vi "Main.vi"() -> ()   [LabVIEW 2023]
uses:
  <vilib>/userDefined/High Color/IMAQdx.ctl
  <vilib>/vision/Image Controls.llb/IMAQ Image.ctl
  <vilib>/vision/driver/NI_Vision_Acquisition_Software.lvlib
  <resource>/objmgr/imaqdx.rc
panel:
  out "New Image":T1
  in  "Object Parameters Attributes":T2={"ReflectedTemperature"=300.0, "AtmosphericTemperature"=300.0, "ExtOpticsTemperature"=300.0, "ObjectEmissivity "=0.95, "RelativeHumidity "=1.0, "ExtOpticsTransmission"=1.0, "EstimatedTransmission"=0.0, "ObjectDistance"=0.0} {"ObjectDistance" min=0.0 max=10000.0 step=1.0; "EstimatedTransmission" min=0.0 max=1.0 step=0.01; "ExtOpticsTransmission" min=0.0 max=1.0 step=0.01; "RelativeHumidity" min=0.0 max=1.0 step=0.01; "ObjectEmissivity" min=0.0 max=1.0 step=0.01; "ExtOpticsTemperature" min=0.0 max=5000.0 step=1.0; "AtmosphericTemperature" min=0.0 max=5000.0 step=1.0; "ReflectedTemperature" min=0.0 max=5000.0 step=1.0}
  in  "PacketSize":u32=1500
  in  "NUCMode":enum16{"Off", "On"}(ring)=enum."On"
  in  "IRFormat":i64(ring)=1 items=["Radiometric", "TemperatureLinear100mK", "TemperatureLinear10mK"]
  in  "Session In":T3
  out "Temperature":dbl(slide) scale=24.600000000000023..25.400000000000034
  out "Image":T1(plugin-control)
  in  "Stop":bool
  # "Please select the camera you want to access the thermal image"
  # "Note: The Image control needs to be set to 16-bit display. This is done by with the following steps\n            1) Right click on the Image display and select 16-Bit Display Mapping to bring up Set 16 Bit Display Mapping window\n            2) Un-tick \"Apply mapping only when Configured bit depth is 0\" in the Set 16 Bit Display Mapping window\n            3) Set the Conversion Method to Full Dynamic if not already selected"
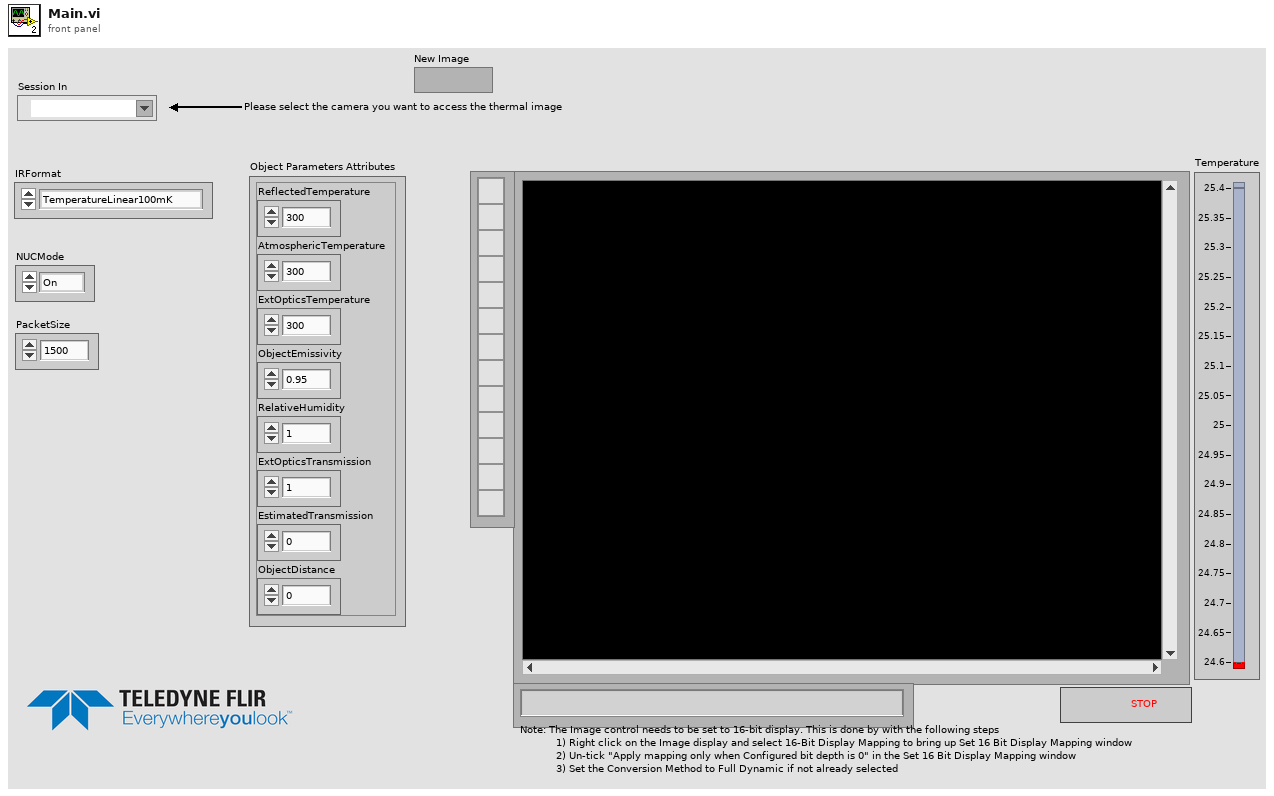
[diagram p1: front panel]
types:
  T1 = typedef "IMAQ Image.ctl" = refnum<image>
  T2 = cluster{"ReflectedTemperature":dbl, "AtmosphericTemperature":dbl, "ExtOpticsTemperature":dbl, "ObjectEmissivity ":dbl, "RelativeHumidity ":dbl, "ExtOpticsTransmission":dbl, "EstimatedTransmission":dbl, "ObjectDistance":dbl}
  T3 = typedef "IMAQdx.ctl" = refnum<k21>
  T4 = typedef "Image Type" = u32
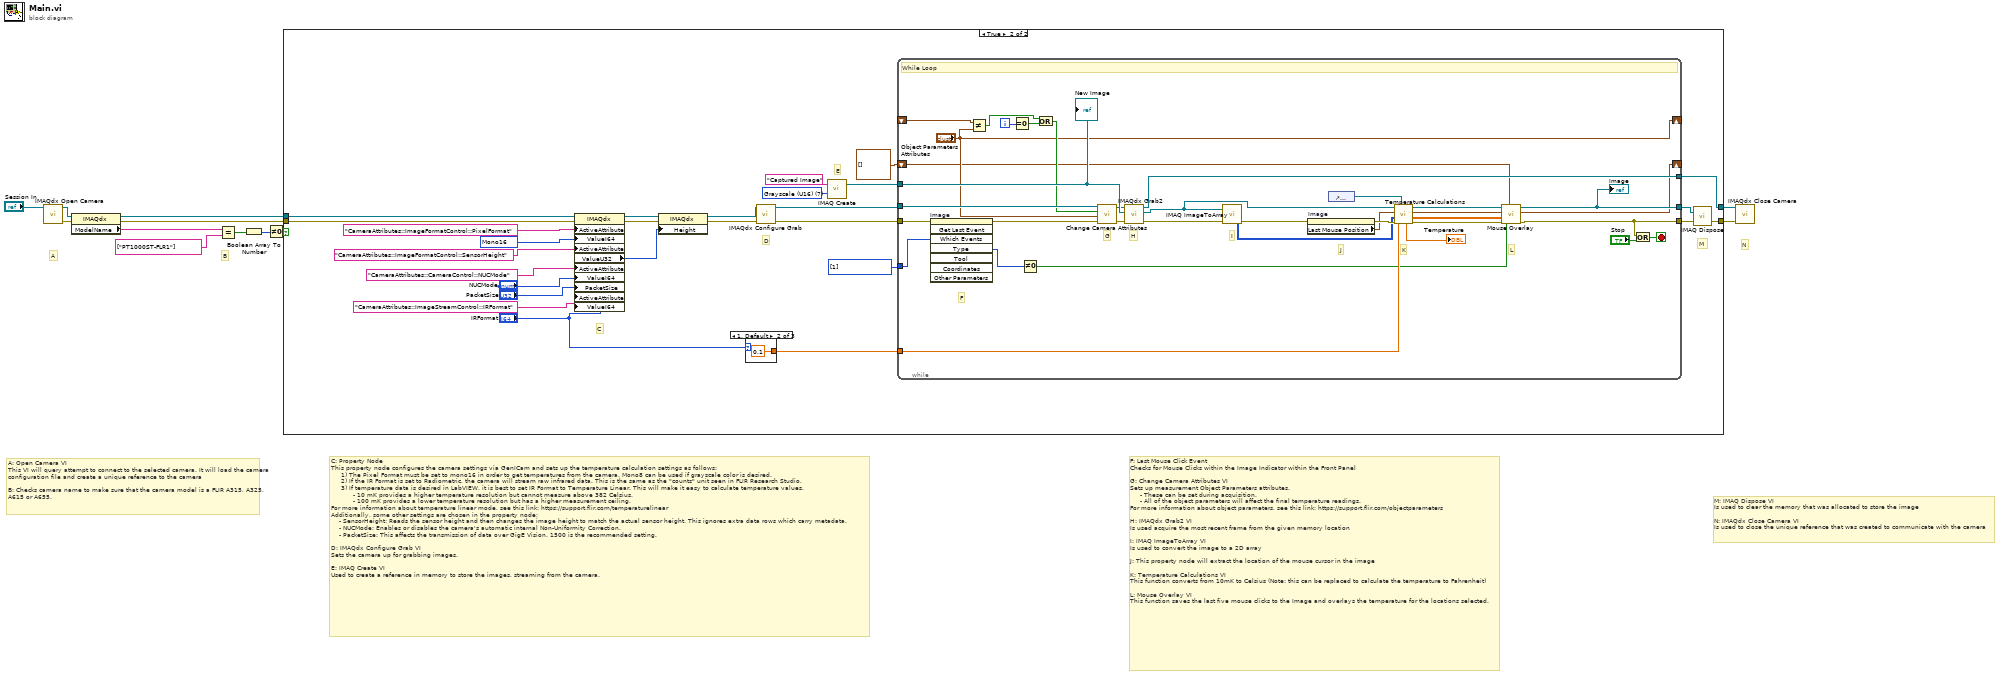
[diagram p0: block diagram]
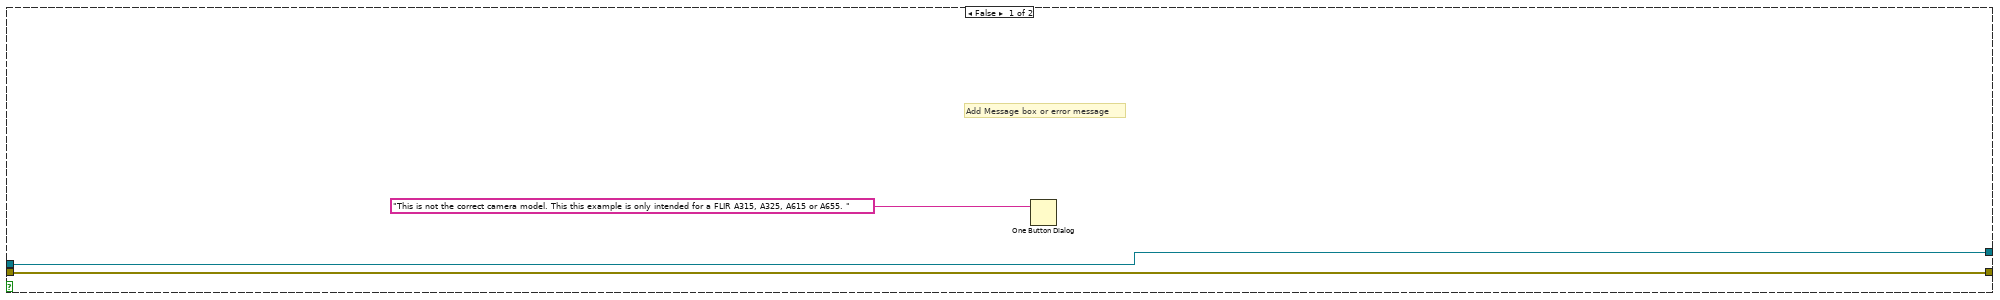
[diagram p2: hidden frame]
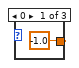
[diagram p3: hidden frame]
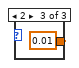
[diagram p4: hidden frame]
diagram:
  # "M: IMAQ Dispose VI\nIs used to clear the memory that was allocated to store the image\n\nN: IMAQdx Close Camera VI\nIs used to close the unique reference that was created to communicate with the camera"
  # "F: Last Mouse Click Event\nChecks for Mouse Clicks within the Image Indicator within the Front Panel \n\nG: Change Camera Attributes VI \nSets up measurement Object Parameters attributes. \n     - These can be set during acquisition. \n     - All of the object parameters will affect the final temperature readings. \nFor more information about object parameters, see this link: https://support.flir.com/objectparameters\n\nH: IMAQdx Grab2 VI\nIs used acquire the most recent frame from the given memory location\n\nI: IMAQ ImageToArray VI\nIs used to convert the image to a 2D array\n\nJ: This property node will extract the location of the mouse cursor in the image\n\nK: Temperature Calculations VI \nThis function converts from 10mK to Celsius (Note: this can be replaced to calculate the temperature to Fahrenheit)\n\nL: Mouse Overlay VI\nThis function saves the last five mouse clicks to the Image and overlays the temperature for the locations selected."
  # "A: Open Camera VI\nThis VI will query attempt to connect to the selected camera. It will load the camera configuration file and create a unique reference to the camera\n\nB: Checks camera name to make sure that the camera model is a FLIR A315, A325, A615 or A655."
  # "B"
  # "N"
  # "A"
  # "C: Property Node\nThis property node configures the camera settings via GenICam and sets up the temperature calculation settings as follows: \n     1) The Pixel Format must be set to mono16 in order to get temperatures from the camera. Mono8 can be used if grayscale color is desired.\n     2) If the IR Format is set to Radiometric, the camera will stream raw infrared data. This is the same as the \"counts\" unit seen in FLIR Research Studio.\n     3) If temperature data is desired in LabVIEW, it is best to set IR Format to Temperature Linear. This will make it easy to calculate temperature values.\n           - 10 mK provides a higher temperature resolution but cannot measure above 382 Celsius.\n           - 100 mK provides a lower temperature resolution but has a higher measurement ceiling.\nFor more information about temperature linear mode, see this link: https://support.flir.com/temperaturelinear\nAdditionally, some other settings are chosen in the property node:\n    - SensorHeight: Reads the sensor height and then changes the image height to match the actual sensor height. This ignores extra data rows which carry metadata.\n    - NUCMode: Enables or disables the camera's automatic internal Non-Uniformity Correction. \n    - PacketSize: This affects the transmission of data over GigE Vision. 1500 is the recommended setting. \n\nD: IMAQdx Configure Grab VI\nSets the camera up for grabbing images.\n\nE: IMAQ Create VI\nUsed to create a reference in memory to store the images, streaming from the camera."
  n1 = call <vilib>:"IMAQdx Open Camera.vi"("Session In"="Session In") -> ("error out"=w8:errorcluster, "Session Out"=w9:T3)  [unwired: 9 in]
  n2 = property class="IMAQdx"(reference=w9, error in=w8) -> (reference out=w7:T3, error out=w6:errorcluster, "ModelName"=w5:string)
  n3 = Equal?(x=w5, y=string[] ["PT1000ST-FLR1"]) -> (x = y?=w2:bool[])
  n4 = Boolean Array To Number(Boolean array=w2) -> (number=w3:u32)
  n5 = Not Equal To 0?(x=w3) -> (x != 0?=w1:bool)
  n6 = case shown="True" w1 {
    tunnel: [w14 w37] -> w11
    tunnel: [w15 w34] -> w10
    tunnel: w7 -> [w15 w33]
    tunnel: w6 -> [w14 w32]
    frame False {
      # "Add Message box or error message"
      n7 = One Button Dialog(message="This is not the correct camera model. This this example is only intended for a FLIR A315, A325, A615 or A655. ") -> ()  [unwired: 1 in, 1 out]
    }
    frame True {
      w30 = i64 17825799 items=["Mono 8"=17301505, "Mono8Signed"=17301506, "Mono10"=17825795, "Mono10Packed"=17563652, "Mono12"=17825797, "Mono12Packed"=17563654, "Mono16"=17825799] ("Ring")
      w40 = T4 7 items=["Grayscale (U8)", "Grayscale (I16)", "Grayscale (SGL)", "Complex (CSG)", "RGB (U32)", "HSL (U32)", "RGB (U64)", "Grayscale (U16)"] ("Image Type")
      w41 = i32[] [1] items=["No Event"=0, "Click Event"=1, "Draw Event"=2, "Size Event"=4, "Scroll Event"=5, "Double Click Event"=8] ("Which Events")
      # "C"
      # "M"
      # "E"
      # "D"
      n8 = property class="IMAQdx"(reference=w33, error in=w32, "ActiveAttribute"="CameraAttributes::ImageFormatControl::PixelFormat", "ValueI64"=w30, "ActiveAttribute"="CameraAttributes::ImageFormatControl::SensorHeight", "ActiveAttribute"="CameraAttributes::CameraControl::NUCMode", "ValueI64"="NUCMode", "PacketSize"="PacketSize", "ActiveAttribute"="CameraAttributes::ImageStreamControl::IRFormat", "ValueI64"="IRFormat") -> (reference out=w21:T3, error out=w19:errorcluster, "ValueU32"=w16:u32)
      n9 = property class="IMAQdx"(reference=w21, error in=w19, "Height"=w16) -> (reference out=w20:T3, error out=w18:errorcluster)
      n10 = case shown="1, Default" "IRFormat" {
        tunnel: [-1.0 0.1 0.01] -> w22
        frame 0 {
        }
        frame 1, Default {
        }
        frame 2 {
        }
      }
      n11 = call <vilib>:"IMAQdx Configure Grab.vi"("error in"=w18, "Session In"=w20) -> ("error out"=w24:errorcluster, "Session Out"=w39:T3)  [unwired: 8 in]
      n12 = call "IMAQ Create"("Image Name"="Captured Image", "Image Type"=w40) -> ("New Image"=w38:T1)  [unwired: 3 in, 1 out]
      n13 = while {
        tunnel: [w58] -> w35
        tunnel: [w57] -> w36
        shift-right: [w56] -> _
        shift-left: cluster{"X":i32, "Y":i32}[] [] ("Array In") -> [w49]
        tunnel: w41 -> [w77]
        tunnel: w39 -> [w73]
        tunnel: w24 -> [w66]
        tunnel: w38 -> [w75]
        tunnel: [w74] -> w34
        tunnel: w22 -> [w60]
        shift-right: ["Object Parameters Attributes"] -> _
        shift-left: _ -> [w55]
        i -> [w70]
        stop <- w80 stop-if-true
        # "L"
        # "K"
        # "I"
        # "H"
        # "G"
        # "F"
        # "J"
        # "While Loop"
        n14 = invoke on="Image" class="ImageControl" method="Get Last Event"(error in=w66, "Which Events"=w77) -> (error out=w65:errorcluster, "Type"=w76:i32)  [unwired: 6 in, 6 out]
        n15 = Not Equal?(x=w55, y="Object Parameters Attributes") -> (x != y?=w68:bool)
        n16 = Equal To 0?(x=w70) -> (x = 0?=w69:bool)
        n17 = Not Equal To 0?(x=w76) -> (x != 0?=w53:bool)
        n18 = Or(x=w68, y=w69) -> (x .or. y?=w67:bool)
        n19 = call "Change Camera Attributes.vi"("error in"=w65, "Object Parameters Attributes"="Object Parameters Attributes", "Boolean"=w67, "Session In"=w73) -> ("error out"=w72:errorcluster, "Session Out"=w71:T3)  [unwired: 6 in]
        n20 = call <vilib>:"IMAQdx Grab2.vi"("error in"=w72, "Image In"=w75, "Session In"=w71) -> ("error out"=w64:errorcluster, "Image Out"=w48:T1, "Session Out"=w74:T3)  [unwired: 5 in, 1 out]
        n21 = call "IMAQ ImageToArray"("error in (no error)"=w64, "Image"=w48) -> ("Image Pixels (U16)"=w62:u16[][], "error out"=w78:errorcluster)  [unwired: 2 in, 3 out]
        n22 = property on="Image" class="ImageControl"(error in=w78) -> (error out=w63:errorcluster, "Last Mouse Position"=w61:cluster{"X":i32, "Y":i32})  [unwired: 1 in, 1 out]
        n23 = control-ref of="Temperature"() -> (w46:refnum<vi>)
        n24 = call "Temperature Calculations.vi"("Conversion"=w60, "Slide Refnum"=w46, "error in"=w63, "Image Pixels (U16)"=w62, "Last Mouse Position:All Elements In"=w61, "Image In"=w48) -> ("error out"=w59:errorcluster, "Temp Array"=w51:dbl[][], "Last Mouse Position:All Elements Out"=w50:cluster{"X":i32, "Y":i32}, "Image Out"=w47:T1, "Temperature"=→"Temperature":dbl)  [unwired: 1 in]
        n25 = call "Mouse Overlay.vi"("Event Occured?"=w53, "Array In"=w49, "error in"=w59, "Temp Array"=w51, "Last Mouse Position:All Elements"=w50, "Image In"=w47) -> ("error out"=w58:errorcluster, "Array Out"=w56:cluster{"X":i32, "Y":i32}[], "Image Out"=w57:T1)  [unwired: 3 in]
        "Image" <- w57
        n26 = Or(x=w58, y="Stop") -> (x .or. y?=w80:bool)
        "New Image" <- w75
      }
      n27 = call "IMAQ Dispose"("Image"=w36, "error in (no error)"=w35) -> ("error out"=w37:errorcluster)  [unwired: 4 in]
    }
  }
  n28 = call <vilib>:"IMAQdx Close Camera.vi"("error in"=w11, "Session In"=w10) -> ()  [unwired: 9 in, 1 out]
